vi "Read.vi"(8 "error in":errorcluster, 11 "TCP in":refnum<k5>) -> (0 "error out":errorcluster, 2 "ASCII QR Code":string, 3 "TCP Network Connection out":refnum<k5>)   [LabVIEW 2023]
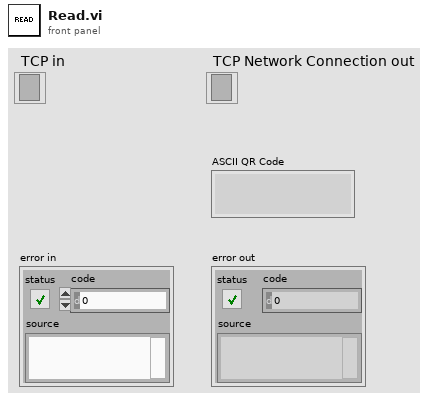
[diagram p1: front panel]
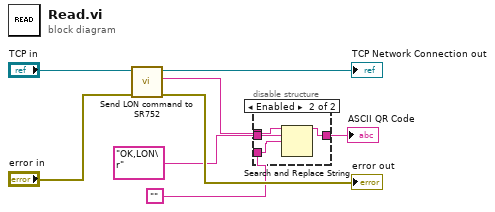
[diagram p0: block diagram]
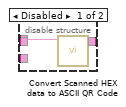
[diagram p2: hidden frame]
diagram:
  n1 = call "Send LON command to SR752.vi"("error in"="error in", "TCP Network Connection in"="TCP in") -> ("error out"=→"error out":errorcluster, "data out"=w8:string, "TCP Network Connection out"=→"TCP Network Connection out":refnum<k5>)  [unwired: 7 in]
  n2 = disable-structure shown="Enabled" {
    disable-tunnel: w8 -> [w10 w14]
    disable-tunnel: [w9 w13] -> w4
    disable-tunnel: "OK,LON\r" -> [_ w12]
    disable-tunnel: "" -> [_ w11]
    frame Disabled {
      n3 = call "Convert Scanned HEX data to ASCII QR Code.vi"("Scanned HEX data"=w10) -> ("ASCII QR Code"=w9:string)  [unwired: 10 in]
    }
    frame Enabled {
      n4 = Search and Replace String(input string=w14, search string=w12, replace string=w11) -> (result string=w13:string)  [unwired: 5 in, 3 out]
    }
  }
  "ASCII QR Code" <- w4
